vi "Noise Reduction.vi"() -> ()   [LabVIEW 2012]
uses:
  <vilib>/picture/picture.llb/Draw 8-Bit Pixmap.vi
  <vilib>/imath/engines/lvmath2/RunTimeEngine/ErrorHandling/NIMS_Finalize Error.vi
  <vilib>/imath/engines/lvmath2/RunTimeEngine/Managers/WorkSpace/UID Generator.vi
  <vilib>/imath/engines/lvmath2/RunTimeEngine/Managers/SymbolTable/Clear UID.vi
  <vilib>/imath/engines/lvmath2/RunTimeEngine/NodeEndStatement/NIMS_NodeEndStatement_Output.vi
  <instcachedir>/0/NIMS_NodeEndStatement_Output_53EC0D466D134D7ABD903AC30B43404B.lvgen/NIMS_NodeEndStatement_Output_53EC0D466D134D7ABD903AC30B43404B_009.vi
  <vilib>/imath/engines/lvmath2/RunTimeEngine/BuiltInFunctions/size/NIMS_I32=size(GM,I32).vi
  <instcachedir>/0/NIMS_I32=size(GM,I32)_25B772E549AD6D489A4AC8DFABEAFFE6.lvgen/NIMS_I32=size(GM,I32)_25B772E549AD6D489A4AC8DFABEAFFE6_006.vi
  <vilib>/imath/engines/lvmath2/RunTimeEngine/BuiltInFunctions/zeros/NIMS_V=zeros(I32,I32).vi
  <vilib>/imath/engines/lvmath2/RunTimeEngine/BuiltInFunctions/hconcatmx/NIMS_hconcatmx.vi
  <instcachedir>/0/NIMS_hconcatmx_918B6D5FBE608C46853AE3202C77FF22.lvgen/NIMS_hconcatmx_918B6D5FBE608C46853AE3202C77FF22_004.vi
  <vilib>/imath/engines/lvmath2/RunTimeEngine/RunTimeType/NIMS_RunTimeType_From StrictType (excl LVString).vi
  <instcachedir>/0/NIMS_RunTimeType_From StrictType (excl LVString)_27CFCE38286AFF43ABD3E48A72A09368.lvgen/NIMS_RunTimeType_From StrictType (excl LVString)_27CFCE38286AFF43ABD3E48A72A09368_000.vi
  <vilib>/imath/engines/lvmath2/RunTimeEngine/ErrorHandling/NIMS_Create Error From Enums.vi
  <vilib>/imath/engines/lvmath2/RunTimeEngine/LocalVariableDefStatement/MC_LocalVariableDefStatement_Display.vi
  <instcachedir>/0/NIMS_I32=size(GM,I32)_25B772E549AD6D489A4AC8DFABEAFFE6.lvgen/NIMS_I32=size(GM,I32)_25B772E549AD6D489A4AC8DFABEAFFE6_005.vi
  <vilib>/imath/engines/lvmath2/RunTimeEngine/BuiltInFunctions/vconcatmx/NIMS_vconcatmx.vi
  <instcachedir>/0/NIMS_vconcatmx_B3FD93D16224B342BBC9BBE24E7F45CD.lvgen/NIMS_vconcatmx_B3FD93D16224B342BBC9BBE24E7F45CD_004.vi
  <vilib>/imath/engines/lvmath2/RunTimeEngine/BuiltInFunctions/size/NIMS_I32Row=size(GM).vi
  <instcachedir>/0/NIMS_I32Row=size(GM)_10ACDCB9F1F84A7E9F42C91D87611FB5.lvgen/NIMS_I32Row=size(GM)_10ACDCB9F1F84A7E9F42C91D87611FB5_006.vi
  <vilib>/imath/engines/lvmath2/RunTimeEngine/BuiltInFunctions/zeros/NIMS_M=zeros(I32V).vi
  <vilib>/imathl/engines/lvmath/Functions/Error Handling/Create Error.vi
  <vilib>/imath/engines/lvmath2/RunTimeEngine/RangeToken/NIMS_Range_R2 - Integer.vi
  <instcachedir>/0/NIMS_Range_R2 - Integer_AAD493E2D93985418B87E485D4769DC2.lvgen/NIMS_Range_R2 - Integer_AAD493E2D93985418B87E485D4769DC2_000.vi
  <vilib>/imath/engines/lvmath2/RunTimeEngine/CommandStatement/MC_CommandStatement_break.vi
  <vilib>/imath/engines/lvmath2/RunTimeEngine/VariableToken/Read/NIMS_Get Elements - SorM(_,_) - Check - Check.vi
  <instcachedir>/0/NIMS_Get Elements - SorM(_,_) - Check - Check_99777BE40F064D4EAE98717AC1B0142A.lvgen/NIMS_Get Elements - SorM(_,_) - Check - Check_99777BE40F064D4EAE98717AC1B0142A_007.vi
  <vilib>/imath/engines/lvmath2/RunTimeEngine/ReplaceToken/NIMS_Replace - Check Row.vi
  <instcachedir>/0/NIMS_Replace - Check Row_72F56154DA6375488AE640E640C52F74.lvgen/NIMS_Replace - Check Row_72F56154DA6375488AE640E640C52F74_005.vi
  <vilib>/imath/engines/lvmath2/RunTimeEngine/ReplaceToken/NIMS_Replace - Check Column.vi
  <instcachedir>/0/NIMS_Replace - Check Column_A3FCF6E68609AF4881EA80658CBF7BA8.lvgen/NIMS_Replace - Check Column_A3FCF6E68609AF4881EA80658CBF7BA8_007.vi
  <vilib>/imath/engines/lvmath2/RunTimeEngine/BuiltInFunctions/median/NIMS_RS=median(RV,I32).vi
  <vilib>/imath/engines/lvmath2/RunTimeEngine/BuiltInFunctions/uint8/NIMS_uint8(real).vi
  <instcachedir>/0/NIMS_uint8(real)_CAA419FBB1354DA296C59E18C46DECF0.lvgen/NIMS_uint8(real)_CAA419FBB1354DA296C59E18C46DECF0_000.vi
  <vilib>/imath/engines/lvmath2/RunTimeEngine/ReplaceToken/NIMS_Replace - Size Check M(_,_)=S.vi
  <instcachedir>/0/NIMS_Replace - Size Check M(_,_)=S_F50CEDB5C64B914DB3C4A1988D778D28.lvgen/NIMS_Replace - Size Check M(_,_)=S_F50CEDB5C64B914DB3C4A1988D778D28_002.vi
  <vilib>/imath/engines/lvmath2/RunTimeEngine/ReplaceToken/NIMS_Replace - M(S,S)=S.vi
  <instcachedir>/0/NIMS_Replace - M(S,S)=S_296BA54965BF82439F001EC285643B20.lvgen/NIMS_Replace - M(S,S)=S_296BA54965BF82439F001EC285643B20_002.vi
  <instcachedir>/0/NIMS_NodeEndStatement_Output_53EC0D466D134D7ABD903AC30B43404B.lvgen/NIMS_NodeEndStatement_Output_53EC0D466D134D7ABD903AC30B43404B_011.vi
  <vilib>/imath/engines/lvmath2/RunTimeEngine/BuiltInFunctions/ones/NIMS_M=ones(I32,I32).vi
  <vilib>/imath/engines/lvmath2/RunTimeEngine/BuiltInFunctions/conv2d/NIMS_conv2d(GM,GM,Str).vi
  <instcachedir>/0/NIMS_conv2d(GM,GM,Str)_C7D81E1B98E043D08C3460674E88E962.lvgen/NIMS_conv2d(GM,GM,Str)_C7D81E1B98E043D08C3460674E88E962_000.vi
  <instcachedir>/0/NIMS_uint8(real)_CAA419FBB1354DA296C59E18C46DECF0.lvgen/NIMS_uint8(real)_CAA419FBB1354DA296C59E18C46DECF0_001.vi
  <vilib>/imath/engines/lvmath2/RunTimeEngine/ErrorHandling/NIMS_Error From Error Code.vi
  <vilib>/imath/engines/lvmath2/RunTimeEngine/Managers/SymbolTable/NIMS_WorkSpace.lvlib
panel:
  in  "Path":path
  out "Median":picture
  out "Flattened":picture
  out "Unflattened":picture
  out "Blurred Image":picture
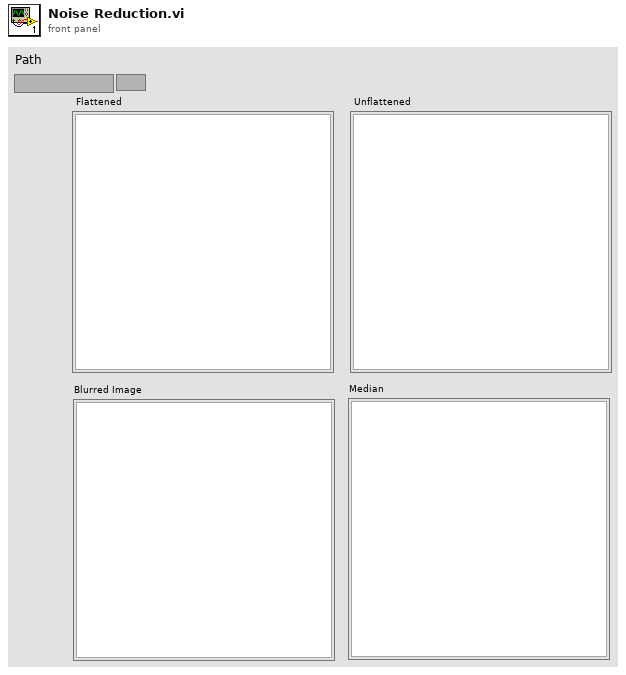
[diagram p1: front panel]
types:
  T1 = typedef "imagedata.ctl" = cluster{"image type":i32, "image depth":i32, "image":u8[], "mask":u8[], "colors":u32[], "Rectangle":cluster{"left":i16, "top":i16, "right":i16, "bottom":i16}}
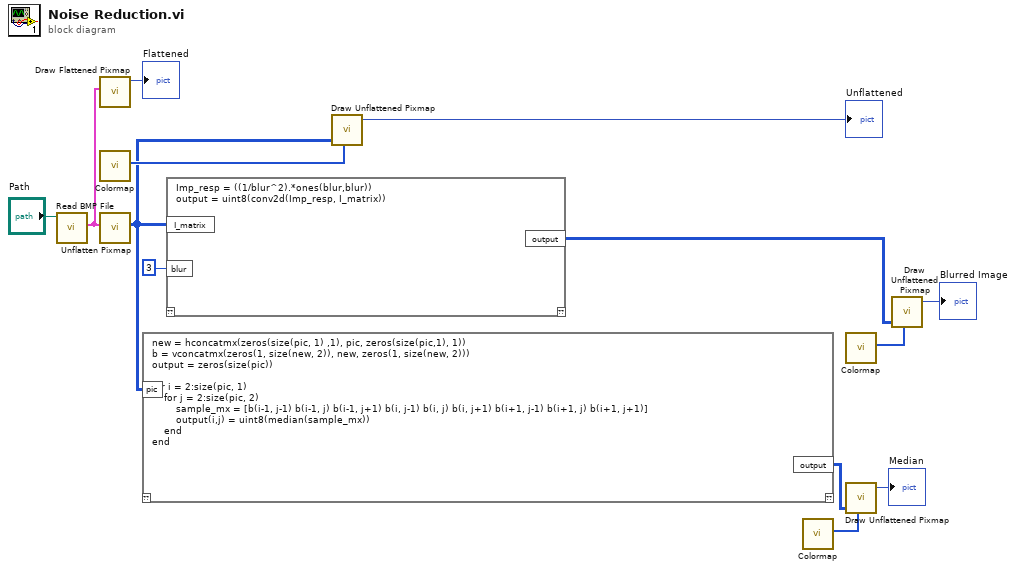
[diagram p0: block diagram]
diagram:
  n1 = call <vilib>:"Read BMP File.vi"("path to BMP file"="Path") -> ("image data"=w10:T1)  [unwired: 8 in, 2 out]
  n2 = call <vilib>:"Draw Flattened Pixmap.vi"("image data"=w10) -> ("new picture"=→"Flattened":picture)  [unwired: 8 in]
  n3 = call "Colormap.vi"() -> ("Array"=w9:u32[])  [unwired: 11 in]
  n4 = call <vilib>:"Unflatten Pixmap.vi"("image data"=w10) -> ("8-bit pixmap"=w5:u8[][])  [unwired: 4 in, 6 out]
  n5 = mathscript code="new = hconcatmx(zeros(size(pic, 1) ,1), pic, zeros(size(pic,1), 1))\nb = vconcatmx(zeros(1, size(new, 2)), new, zeros(1, size(new, 2)))\noutput = zeros(size(pic))\n\nfor i = 2:size(pic, 1)\n    for j = 2:size(pic, 2)\n        sample_mx = [b(i-1, j-1) b(i-1, j) b(i-1, j+1) b(i, j-1) b(i, j) b(i, j+1) b(i+1, j-1) b(i+1, j) b(i+1, j+1)]\n        output(i,j) = uint8(median(sample_mx))\n    end\nend"("pic"=w5) -> ("output"=w1:i32[][])  [unwired: 1 in, 1 out]
  n6 = mathscript code="Imp_resp = ((1/blur^2).*ones(blur,blur))\noutput = uint8(conv2d(Imp_resp, I_matrix))"("I_matrix"=w5, "blur"=3) -> ("output"=w11:u8[][])  [unwired: 1 in, 1 out]
  n7 = call-poly <vilib>:"Draw Unflattened Pixmap.vi"("data"=w5, "color table"=w9) -> ("new picture"=→"Unflattened":picture)  [unwired: 7 in]
  n8 = call "Colormap.vi"() -> ("Array"=w4:u32[])  [unwired: 11 in]
  n9 = call "Colormap.vi"() -> ("Array"=w13:u32[])  [unwired: 11 in]
  n10 = call-poly <vilib>:"Draw Unflattened Pixmap.vi"("data"=w1, "color table"=w4) -> ("new picture"=→"Median":picture)  [unwired: 7 in]
  n11 = call-poly <vilib>:"Draw Unflattened Pixmap.vi"("data"=w11, "color table"=w13) -> ("new picture"=→"Blurred Image":picture)  [unwired: 7 in]
